vi "Set ILC.vi"(10 "ILC":refnum<class "FAILC.lvclass">, 11 "Model in":refnum<class "Model.lvclass">) -> (3 "Model out":refnum<class "Model.lvclass">)   [LabVIEW 2015, in "Model.lvclass"]
uses:
  Model.lvclass
  Common_RT_FAILC/FAILC/FAILC.lvclass
  Model.lvclass/Model.ctl
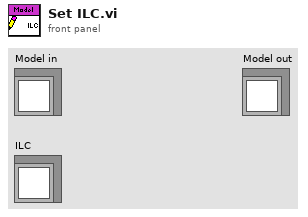
[diagram p1: front panel]
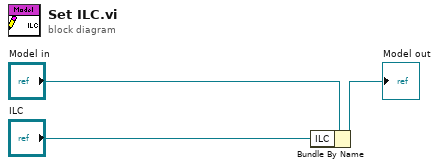
[diagram p0: block diagram]
diagram:
  n1 = Bundle By Name(cluster="Model in", "ILC"="ILC") -> (→"Model out":refnum<class "Model.lvclass">)
